vi "CallEdge_Create.vi"(0 "reference":refnum<class "CallEdge.lvclass">, 5 "error in (no error)":errorcluster) -> (14 "reference out":refnum<class "CallEdge.lvclass">, 16 "# of objects":i32, 19 "error out":errorcluster)   [LabVIEW 2012, in "CallEdge.lvclass"]
doc: "Creates and initializes a new CallEdge object.\n\nThis object should be destroyed using a CallEdge destructor VI or a virtual base class destructor VI.\n\n[GOOP 2.3]"
uses:
  <resource>/Framework/Providers/Open_GDS/UML/CallEdge_class/CallEdge.lvclass
  <resource>/Framework/Providers/Open_GDS/UML/SegmentedLineEdge_class/SegmentedLineEdge.lvclass
panel:
  # "The input reference should only\nbe wired when this method is called\nby a sub class constructor."
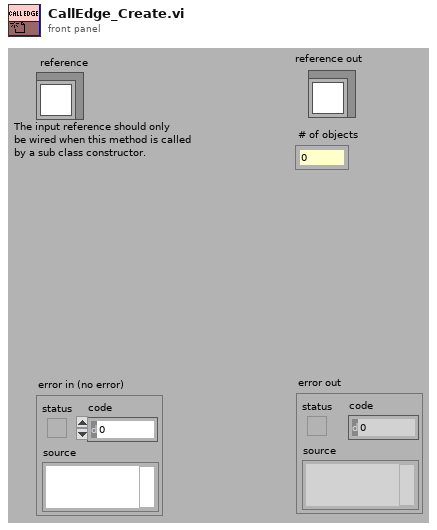
[diagram p1: front panel]
types:
  T1 = typedef "CallEdge.lvclass/ObjectAttributes.ctl" = cluster{"signal":bool}
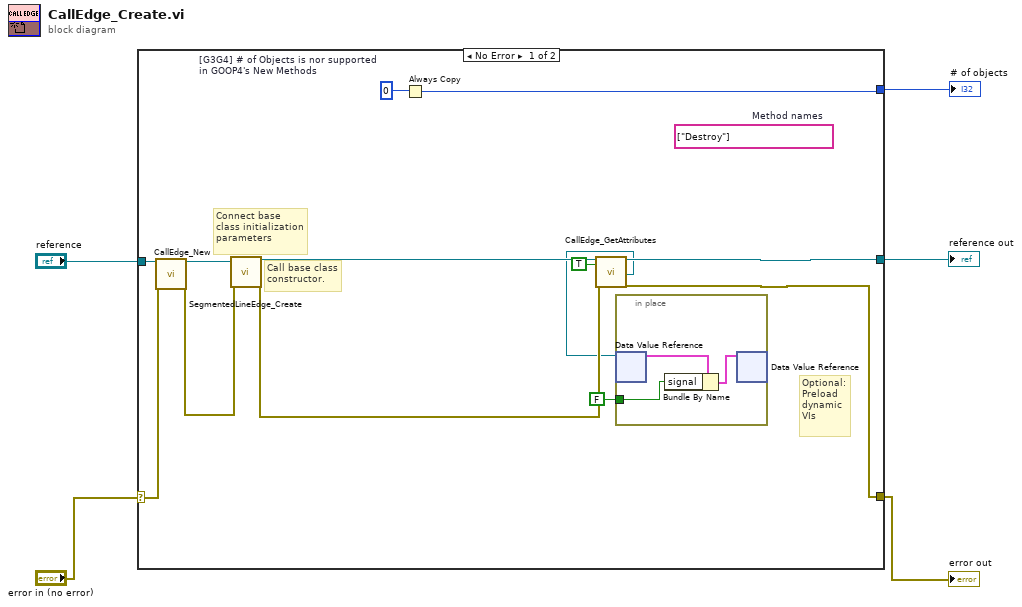
[diagram p0: block diagram]
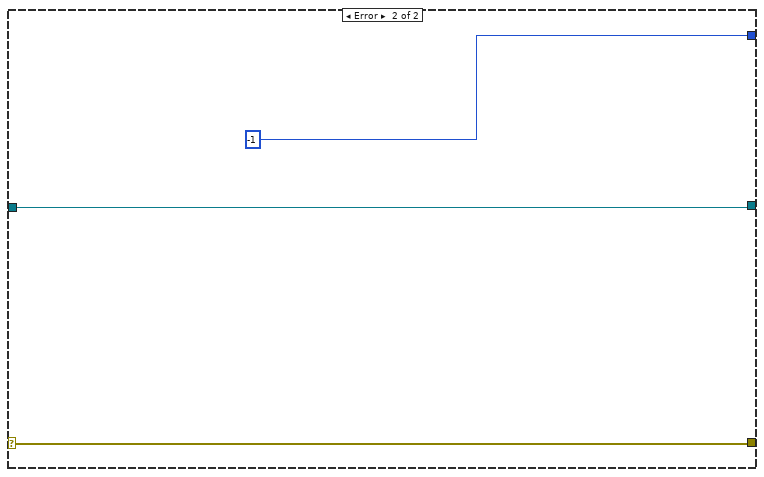
[diagram p2: hidden frame]
diagram:
  n1 = case shown="No Error" "error in (no error)" {
    selector: "error in (no error)" -> [w18 w23]
    tunnel: [w12 w22] -> w5
    tunnel: [w11 w23] -> w4
    tunnel: [w10 -1 ("Nr of open handles")] -> w3
    tunnel: "reference" -> [w17 w22]
    frame No Error {
      w6 = 0  # [G3G4] # of Objects is nor supported in GOOP4's New Methods
      (unwired) string[] ["Destroy"]  # Method names
      # "Optional:\nPreload\ndynamic\nVIs"
      # "Connect base\nclass initialization\nparameters"
      # "Call base class\nconstructor."
      n2 = call <resource>:"CallEdge_New.vi"("reference in"=w17, "error in (no error)"=w18) -> ("reference out"=w14:refnum<class "CallEdge.lvclass">, "error out"=w16:errorcluster)  [unwired: 2 in, 14 out]
      n3 = call <resource>:"SegmentedLineEdge_Create.vi"("reference"=w14, "error in (no error)"=w16) -> ("reference out"=w13:refnum<class "CallEdge.lvclass">, "error out"=w15:errorcluster)  [unwired: 1 in, 15 out]
      n4 = Always Copy(1:w6) -> (0:w10:i32)
      n5 = call <resource>:"CallEdge_GetAttributes.vi"("reference in"=w13, "OnlyGetDvrReference(False)"=TRUE, "error in (no error)"=w15) -> ("reference out"=w12:refnum<class "CallEdge.lvclass">, "DataRef"=w8:refnum<data-value>, "error out"=w11:errorcluster)  [unwired: 13 in, 1 out]
      n6 = in-place {
        in-place-border: FALSE ("signal") -> [w20]
        n7 = in-place-dvr #1(w8) -> (w21:T1)  [unwired: 1 out]
        n8 = Bundle By Name(cluster=w21, "signal"=w20) -> (w19:T1)
        n9 = in-place-dvr #1(w19) -> ()  [unwired: 2 out]
      }
    }
    frame Error {
    }
  }
  "error out" <- w4
  "reference out" <- w5
  "# of objects" <- w3
